vi "LCD Scrolling Text Display.vi"() -> ()   [LabVIEW 2021]
uses:
  <extravilib>/ChannelInstances/Stream-str/Read With Abort.vi
  <extravilib>/ChannelInstances/Tag-u32/Write With Abort.vi
  <extravilib>/ChannelInstances/Tag-bool/Write With Abort.vi
  <extravilib>/ChannelInstances/Stream-str/EndpointRead.vi
  <extravilib>/ChannelInstances/Tag-u32/Instantiate.vi
  <extravilib>/ChannelInstances/Stream-str/Instantiate.vi
  <extravilib>/ChannelInstances/Stream-str/)Channel.vi
  <resource>/ChannelSupport/_ChannelSupport/WaitIfNeeded.vi
  <extravilib>/ChannelInstances/Tag-bool/Instantiate.vi
  <extravilib>/ChannelInstances/Tag-u32/Endpoint.vi
  <extravilib>/ChannelInstances/Tag-bool/Endpoint.vi
  <extravilib>/ChannelInstances/Tag-bool.lvlib
  <extravilib>/ChannelInstances/Tag-u32.lvlib
  <extravilib>/ChannelInstances/Stream-str.lvlib
panel:
  in  "Scroll Interval":u32=250
  out "LCD Display":string
  in  "Stop":bool
  in  "LCD Displayable Characters Number":u8=16
  in  "String To Display:":string="Made using LabVIEW"
  # "Set before program start"
  # "Settable during program run"
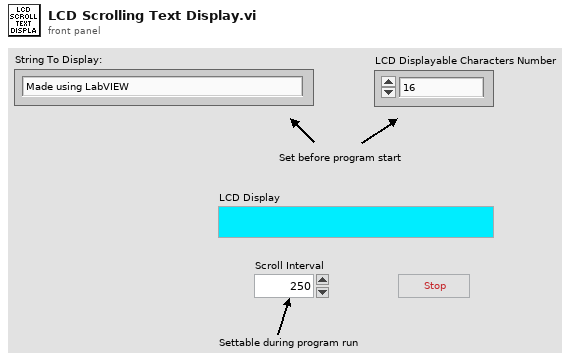
[diagram p1: front panel]
types:
  T1 = typedef "Tag-u32.lvlib/))Channel.ctl" = refnum<queue>
  T2 = typedef "Tag-bool.lvlib/))Channel.ctl" = refnum<queue>
  T3 = typedef "Stream-str.lvlib/)Channel.ctl" = refnum<queue>
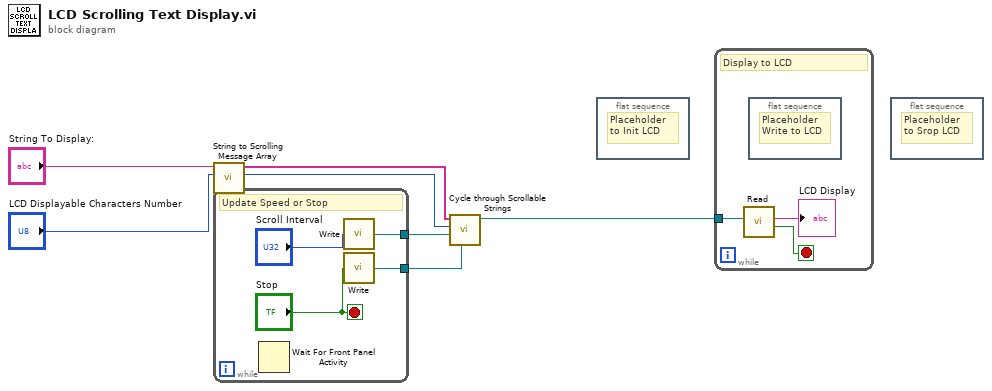
[diagram p0: block diagram]
diagram:
  n1 = call "String to Scrolling Message Array.vi"("LCD Displayable Characters Number"="LCD Displayable Characters Number", "String To Display:"="String To Display:") -> ("Scrollable Messages Array Size"=w1:i32, "Scrolling Messages Array"=w3:string[])  [unwired: 8 in]
  n2 = while {
    tunnel: [w11] -> w5
    tunnel: [w9] -> w2
    stop <- "Stop" stop-if-true
    # "Update Speed or Stop"
    n3 = Wait For Front Panel Activity() -> ()  [unwired: 3 in, 1 out]
    n4 = call <extravilib>:"Write.vi"("element"="Scroll Interval") -> ("channel"=w9:T1)  [unwired: 1 out]
    n5 = call <extravilib>:"Write.vi"("element"="Stop") -> ("channel"=w11:T2)  [unwired: 1 out]
  }
  n6 = call "Cycle through Scrollable Strings.vi"("Stop?"=w5, "Scroll Interval"=w2, "Scrollable Messages Array Size"=w1, "Scrolling Messages Array"=w3) -> ("String to Display"=w4:T3)  [unwired: 7 in]
  n7 = flat-sequence {
    frame #0 {
      # "Placeholder to Init LCD"
    }
  }
  n8 = while {
    tunnel: w4 -> [w14]
    stop <- w12 stop-if-true
    # "Display to LCD"
    n9 = call <extravilib>:"Read.vi"("channel"=w14) -> ("last element?"=w12:bool, "element"=→"LCD Display":string)  [unwired: 6 in, 3 out]
    n10 = flat-sequence {
      frame #0 {
        # "Placeholder Write to LCD"
      }
    }
  }
  n11 = flat-sequence {
    frame #0 {
      # "Placeholder to Srop LCD"
    }
  }
